vi "Units_FeetToMeters.vi"(10 "Feet":dbl) -> (2 "Meters":dbl)   [LabVIEW 2019, in "Trajectory_Library.lvlib"]
doc: "Convert Meters to Feet"
uses:
  Trajectory_Library.lvlib
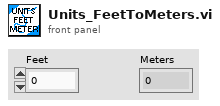
[diagram p1: front panel]
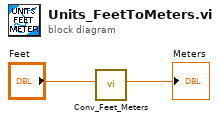
[diagram p0: block diagram]
diagram:
  n1 = call "Conv_Feet_Meters.vi"("Feet"="Feet") -> ("Meters"=→"Meters":dbl)  [unwired: 10 in]
